vi "IsDiabled.vi"() -> (3 "Is Disabled?":bool)   [LabVIEW 2014]
uses:
  <vilib>/Rock Robotics/WPI/DriverStation/WPI_DriverStationRobotMode2.ctl
  Robot Global Data.vi
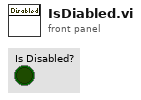
[diagram p1: front panel]
types:
  T1 = typedef "WPI_DriverStationRobotMode2.ctl" = enum16{"Autonomous Disabled", "Autonomous Enabled", "Teleop Disabled", "Teleop Enabled", "Disconnected", "Finish", "Test Disabled", "Test Enabled"}
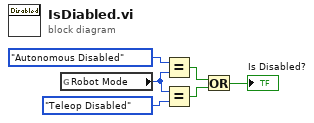
[diagram p0: block diagram]
diagram:
  n1 = global read "Robot Global Data.vi" "Robot Mode"() -> (w4:T1)
  n2 = Equal?(x=WPI_DriverStationRobotMode2."Autonomous Disabled" ("Robot Mode"), y=w4) -> (x = y?=w2:bool)
  n3 = Equal?(x=w4, y=WPI_DriverStationRobotMode2."Teleop Disabled" ("Robot Mode")) -> (x = y?=w5:bool)
  n4 = Or(x=w2, y=w5) -> (x .or. y?=→"Is Disabled?":bool)
